vi "Prepare SV Libraries.vi"(8 "error in (no error)":errorcluster, 11 "SV B-M in":refnum<class "SV B-M (Host).lvclass">) -> (0 "error out":errorcluster, 3 "SV B-M out":refnum<class "SV B-M (Host).lvclass">)   [LabVIEW 2015, in "SV B-M (Host).lvclass"]
doc: "From a group of prebuilt SV libraries, gather all the necessary libraries of the correct size and data type to execute this particular test. Place these libraries in the directory for this particular sequence."
uses:
  SV B-M (Host).lvclass
  SV B-M (Host).lvclass/SV B-M (Host).ctl
  Listbox - In Progress.vi
  Listbox - Complete.vi
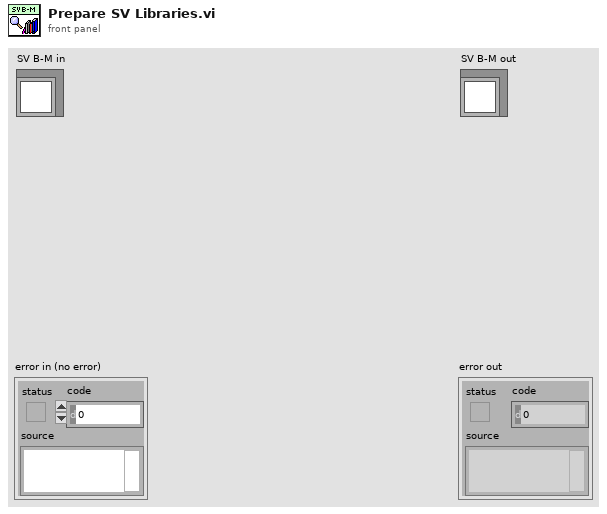
[diagram p1: front panel]
types:
  T1 = enum32{"invalid app kind", "Development System", "Run Time System", "Student Edition", "Embedded LabVIEW", "Evaluation", "Custom"}
  T2 = typedef "Variable Data Type.ctl" = enum16{"U8", "U16", "U32", "U64", "I8", "I16", "I32", "I64", "Single", "Double", "Boolean", "String"}
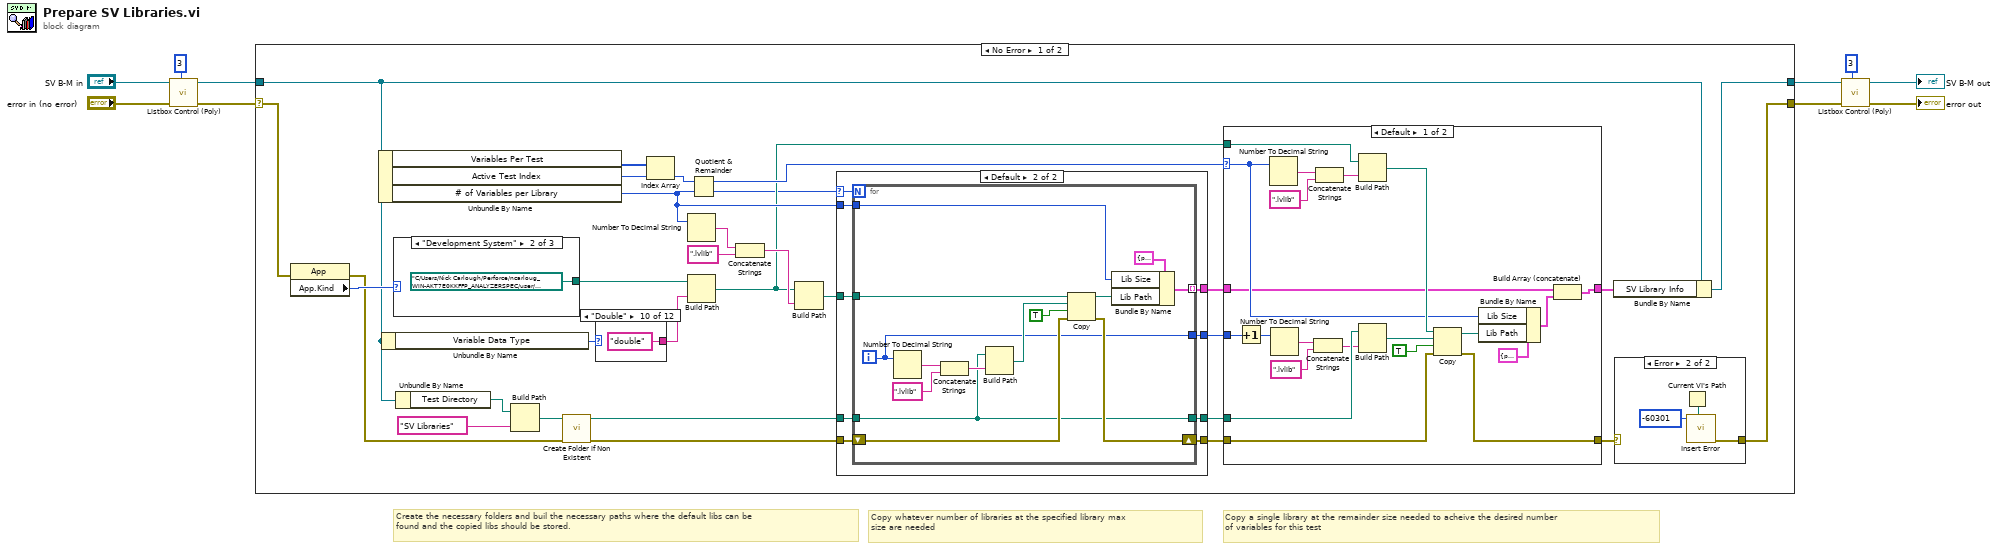
[diagram p0: block diagram]
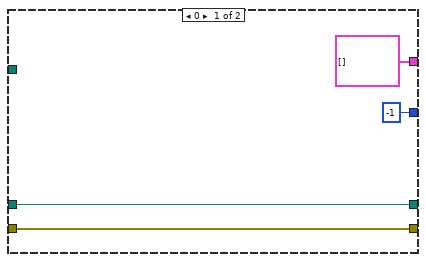
[diagram p3: hidden frame]
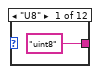
[diagram p5: hidden frame]
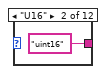
[diagram p6: hidden frame]
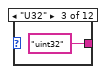
[diagram p7: hidden frame]
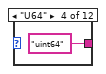
[diagram p8: hidden frame]
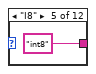
[diagram p9: hidden frame]
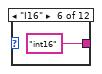
[diagram p10: hidden frame]
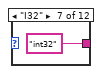
[diagram p11: hidden frame]
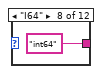
[diagram p12: hidden frame]
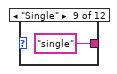
[diagram p13: hidden frame]
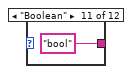
[diagram p14: hidden frame]
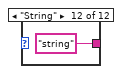
[diagram p15: hidden frame]
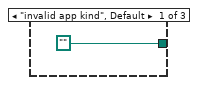
[diagram p16: hidden frame]
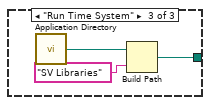
[diagram p17: hidden frame]
diagram:
  # "Copy a single library at the remainder size needed to acheive the desired number\nof variables for this test"
  # "Copy whatever number of libraries at the specified library max\nsize are needed"
  # "Create the necessary folders and buil the necessary paths where the default libs can be\nfound and the copied libs should be stored."
  n1 = call-poly "Listbox Control (Poly).vi"("Row to Update"=3, "error in (no error)"="error in (no error)", "SV B-M In"="SV B-M in") -> ("error out"=w7:errorcluster, "SV B-M Out"=w9:refnum<class "SV B-M (Host).lvclass">)  [unwired: 7 in]
  n2 = case shown="No Error" w7 {
    selector: w7 -> [w17 w113]
    tunnel: w9 -> [w16 w114]
    tunnel: [w14 w114] -> w4
    tunnel: [w11 w113] -> w3
    frame No Error {
      n3 = property class="App"(error in=w17) -> (error out=w32:errorcluster, "App.Kind"=w41:T1)  [unwired: 1 in, 1 out]
      n4 = Unbundle By Name(w16) -> ("Variables Per Test"=w40:u32[], "Active Test Index"=w39:i32, "# of Variables per Library"=w24:u16)
      n5 = Unbundle By Name(w16) -> ("Variable Data Type"=w38:T2)
      n6 = case shown="\"Development System\"" w41 {
        tunnel: [path "" path "C:/Users/Nick Carlough/Perforce/ncarloug_WIN-AKT7E0KKFFP_ANALYZERSPEC/user/ncarloug/Shared Variable Benchmarking Utility/builds/Windows Host/SV Libraries" w110] -> w37
        frame "invalid app kind", Default {
        }
        frame "Development System" {
        }
        frame "Run Time System" {
          n7 = call <vilib>:"Application Directory.vi"() -> ("Application Directory"=w112:path)
          n8 = Build Path(base path=w112, name or relative path="SV Libraries") -> (appended path=w110:path)
        }
      }
      n9 = Unbundle By Name(w16) -> ("Test Directory"=w34:path)
      n10 = Build Path(base path=w34, name or relative path="SV Libraries") -> (appended path=w33:path)
      n11 = call "Create Folder if Non Existent.vi"("error in (no error)"=w32, "Folder to Create"=w33) -> ("error out"=w30:errorcluster, "New Path Out"=w25:path)  [unwired: 8 in]
      n12 = case shown="\"Double\"" w38 {
        tunnel: ["uint8" "uint16" "uint32" "uint64" "int8" "int16" "int32" "int64" "single" "double" "bool" "string"] -> w36
        frame "U8" {
        }
        frame "U16" {
        }
        frame "U32" {
        }
        frame "U64" {
        }
        frame "I8" {
        }
        frame "I16" {
        }
        frame "I32" {
        }
        frame "I64" {
        }
        frame "Single" {
        }
        frame "Double" {
        }
        frame "Boolean" {
        }
        frame "String" {
        }
      }
      n13 = Index Array(array=w40, index=w39) -> (element=w31:u32)
      n14 = Number To Decimal String(number=w24) -> (decimal integer string=w29:string)  [unwired: 1 in]
      n15 = Build Path(base path=w37, name or relative path=w36) -> (appended path=w19:path)
      n16 = Quotient & Remainder(x=w31, y=w24) -> (x-y*floor(x/y)=w23:u32, floor(x/y)=w13:u32)
      n17 = Concatenate Strings(w29, ".lvlib") -> (w27:string)
      n18 = Build Path(base path=w19, name or relative path=w27) -> (appended path=w26:path)
      n19 = case shown="Default" w13 {
        selector: w13 -> [_ w50]
        tunnel: w30 -> [w46 w58]
        tunnel: w26 -> [_ w57]
        tunnel: w25 -> [w47 w56]
        tunnel: w24 -> [_ w55]
        tunnel: [cluster{"Lib Path":path, "Lib Size":u16}[] [] w54] -> w22
        tunnel: [-1 w53] -> w21
        tunnel: [w47 w52] -> w20
        tunnel: [w46 w51] -> w18
        frame 0 {
        }
        frame Default {
          n20 = for {
            N: w50 -> [_]
            shift-right: [w61] -> w51
            shift-left: w58 -> [w68]
            tunnel: w57 -> [w71]
            tunnel: w56 -> [w59]
            tunnel: w55 -> [w63]
            tunnel: [w62] -> w54 mode=indexing
            tunnel: [w60] -> w53
            tunnel: [w59] -> w52
            i -> [w60]
            n21 = Number To Decimal String(number=w60) -> (decimal integer string=w67:string)  [unwired: 1 in]
            n22 = Concatenate Strings(w67, ".lvlib") -> (w72:string)
            n23 = Build Path(base path=w59, name or relative path=w72) -> (appended path=w70:path)
            n24 = Copy(8:w68, 9:TRUE, 10:w70, 11:w71) -> (0:w61:errorcluster, 3:w64:path)  [unwired: 1 in, 1 out]
            n25 = Bundle By Name(cluster=cluster{"Lib Path":path, "Lib Size":u16} {"Lib Path"=path "", "Lib Size"=0}, "Lib Size"=w63, "Lib Path"=w64) -> (w62:cluster{"Lib Path":path, "Lib Size":u16})
          }
        }
      }
      n26 = case shown="Default" w23 {
        selector: w23 -> [w77 _]
        tunnel: w22 -> [w75 w95]
        tunnel: w21 -> [w93 _]
        tunnel: w20 -> [w91 _]
        tunnel: w19 -> [w84 _]
        tunnel: w18 -> [w81 w94]
        tunnel: [w76 w94] -> w12
        tunnel: [w73 w95] -> w15
        frame Default {
          n27 = Increment(x=w93) -> (x+1=w92:i32)
          n28 = Number To Decimal String(number=w77) -> (decimal integer string=w87:string)  [unwired: 1 in]
          n29 = Number To Decimal String(number=w92) -> (decimal integer string=w90:string)  [unwired: 1 in]
          n30 = Concatenate Strings(w90, ".lvlib") -> (w88:string)
          n31 = Concatenate Strings(w87, ".lvlib") -> (w85:string)
          n32 = Build Path(base path=w84, name or relative path=w85) -> (appended path=w82:path)
          n33 = Build Path(base path=w91, name or relative path=w88) -> (appended path=w83:path)
          n34 = Copy(8:w81, 9:TRUE, 10:w83, 11:w82) -> (0:w76:errorcluster, 3:w78:path)  [unwired: 1 in, 1 out]
          n35 = Bundle By Name(cluster=cluster{"Lib Path":path, "Lib Size":u16} {"Lib Path"=path "", "Lib Size"=0}, "Lib Size"=w77, "Lib Path"=w78) -> (w74:cluster{"Lib Path":path, "Lib Size":u16})
          n36 = Build Array (concatenate)(w75, w74) -> (w73:cluster{"Lib Path":path, "Lib Size":u16}[])
        }
        frame 0 {
        }
      }
      n37 = Bundle By Name(cluster=w16, "SV Library Info"=w15) -> (w14:refnum<class "SV B-M (Host).lvclass">)
      n38 = case shown="Error" w12 {
        selector: w12 -> [w42 _]
        tunnel: [w42 w45] -> w11
        frame No Error {
        }
        frame Error {
          n39 = Current VI's Path() -> (path=w43:path)
          n40 = call "Insert Error.vi"("VI Path"=w43, "Error Code"=-60301) -> ("error out"=w45:errorcluster)  [unwired: 9 in]
        }
      }
    }
    frame Error {
    }
  }
  n41 = call-poly "Listbox Control (Poly).vi"("Row to Update"=3, "error in (no error)"=w3, "SV B-M In"=w4) -> ("error out"=→"error out":errorcluster, "SV B-M Out"=→"SV B-M out":refnum<class "SV B-M (Host).lvclass">)  [unwired: 7 in]
